vi "Target OS Specific Channels.vi"(8 "error in (no error)":errorcluster, 11 "Device Item Ref in":T1 format="%.0x") -> (0 "error out":errorcluster, 3 "Item Ref out":T1 format="%.0x")   [LabVIEW 2018, in "Chassis TimeSync System Explorer.lvlib"]
uses:
  Chassis TimeSync System Explorer.lvlib
  <vilib>/NI Veristand/Custom Device API/Custom Device Item Ref.ctl
  <vilib>/NI Veristand/Custom Device API/Custom Device Channel Type.ctl
  Shared/Constants.vi
  <vilib>/NI Veristand/Custom Device API/Custom Device API.lvlib
  Shared/Chassis TimeSync Shared.lvlib
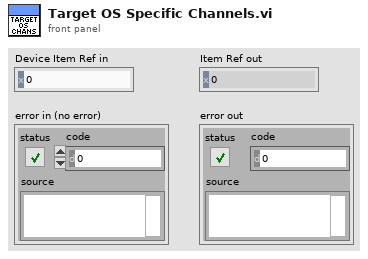
[diagram p1: front panel]
types:
  T1 = typedef "Custom Device API.lvlib/Custom Device Item Ref.ctl" = u64
  T2 = typedef "Custom Device API.lvlib/Custom Device Target Type.ctl" = enum16{"PharLap", "VxWorks", "Windows", "Linux_32_ARM", "Linux_x64"}
  T3 = typedef "Custom Device API.lvlib/Custom Device Channel Type.ctl" = enum16{"Input", "Output"}
  T4 = typedef "Chassis TimeSync Shared.lvlib/Channel.ctl" = cluster{"Name":string, "Units":string, "Default":dbl, "Description":string}
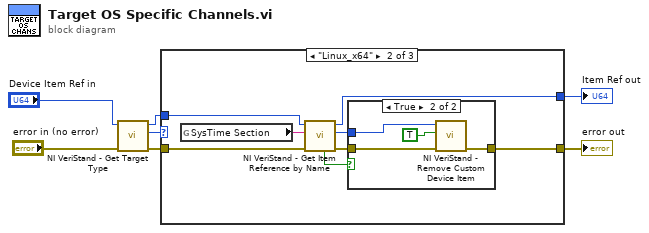
[diagram p0: block diagram]
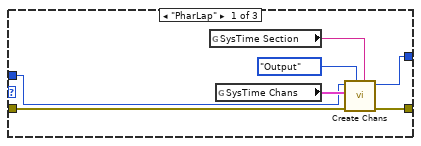
[diagram p2: hidden frame]
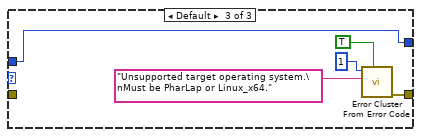
[diagram p4: hidden frame]
diagram:
  n1 = call <vilib>:"NI VeriStand - Get Target Type.vi"("error in (no error)"="error in (no error)", "Item Ref in"="Device Item Ref in") -> ("error out"=w2:errorcluster, "Target Type"=w6:T2, "Item Ref out"=w1:T1)  [unwired: 7 in]
  n2 = case shown="\"Linux_x64\"" w6 {
    tunnel: [w11 w17 w32] -> w3
    tunnel: [w10 w20 w28] -> w4
    tunnel: w2 -> [w8 w22 _]
    tunnel: w1 -> [w9 w21 w28]
    frame "PharLap" {
      n3 = global read "Constants.vi" "SysTime Section"() -> (w12:string)
      n4 = global read "Constants.vi" "SysTime Chans"() -> (w14:T4[])
      n5 = call "Create Chans.vi"("New Section Name (none)"=w12, "Type"=Custom_Device_Channel_Type."Output", "error in (no error)"=w8, "Channels"=w14, "Section Ptr"=w9) -> ("error out"=w11:errorcluster, "Section Ptr dup"=w10:T1)  [unwired: 5 in]
    }
    frame "Linux_x64" {
      n6 = global read "Constants.vi" "SysTime Section"() -> (w15:string)
      n7 = call <vilib>:"NI VeriStand - Get Item Reference by Name.vi"("error in (no error)"=w22, "Item Name"=w15, "Parent Ref in"=w21) -> ("error out"=w19:errorcluster, "Item Ref"=w18:T1, "Parent Ref out"=w20:T1, "Found"=w16:bool)  [unwired: 5 in]
      n8 = case shown="True" w16 {
        tunnel: w19 -> [w23 w27]
        tunnel: w18 -> [_ w25]
        tunnel: [w23 w24] -> w17
        frame False {
        }
        frame True {
          n9 = call <vilib>:"NI VeriStand - Remove Custom Device Item.vi"("error in (no error)"=w27, "Force Delete (F)"=TRUE, "Item Ref in"=w25) -> ("error out"=w24:errorcluster)  [unwired: 7 in, 1 out]
        }
      }
    }
    frame Default {
      n10 = call <vilib>:"Error Cluster From Error Code.vi"("show call chain? (False)"=TRUE, "error message (\"\")"="Unsupported target operating system.\nMust be PharLap or Linux_x64." ("error message (\"\")"), "error code (0)"=1) -> ("error out"=w32:errorcluster)  [unwired: 6 in]
    }
  }
  "Item Ref out" <- w4
  "error out" <- w3
